vi "Read configuration.vi"(8 "error in":errorcluster, 11 "Cfg Channel in":refnum<class "Cfg Channel.lvclass">) -> (0 "error out":errorcluster, 2 "configuration":refnum<class "NISE_CEF_serializable configuration.lvclass">, 3 "Cfg Channel out":refnum<class "Cfg Channel.lvclass">)   [LabVIEW 2013, in "Cfg Channel.lvclass"]
uses:
  Cfg Channel.lvclass
  CEF_TreeControl/serializable configuration/NISE_CEF_serializable configuration.lvclass
  Cfg Channel.lvclass/Cfg Channel.ctl
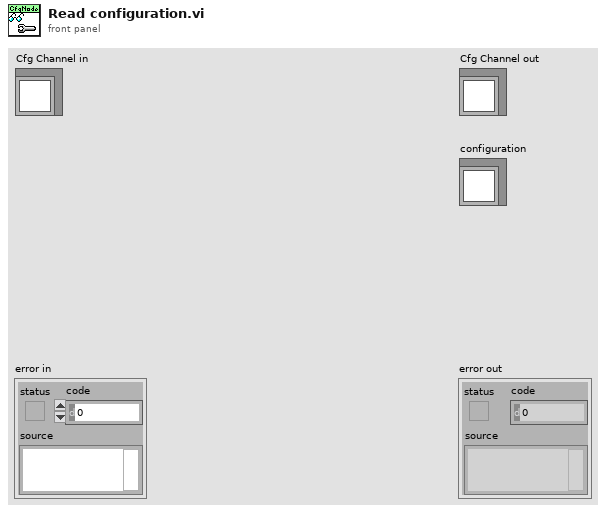
[diagram p1: front panel]
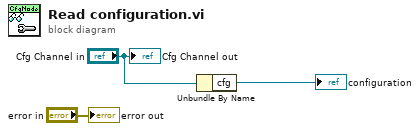
[diagram p0: block diagram]
diagram:
  n1 = Unbundle By Name("Cfg Channel in") -> ("cfg"=→"configuration":refnum<class "channel config object.lvclass">)
  "error out" <- "error in"
  "Cfg Channel out" <- "Cfg Channel in"
